vi "Localization FGV.vi"(0 "Action":T1, 1 "Dictionary File Path":path, 5 "VI in":refnum<vi>, 7 "Target Language":string, 9 "UID":string, 11 "error in":errorcluster) -> (6 "Dictionary":T2, 8 "Languages":string[](array[string]), 10 "Translated Word":string, 14 "Current Language":string, 15 "error out":errorcluster)   [LabVIEW 2017, in "JKI Simple Localization.lvlib"]
uses:
  API/JKI Simple Localization.lvlib
  Definitions/Dictionary--Cluster.ctl
  Definitions/Private/Font -- Cluster.ctl
  Definitions/Private/Phrase Dictionary Entry -- Cluster.ctl
  Definitions/Private/Localization FGV Action -- Enum.ctl
  Definitions/Private/VI Info -- Cluster.ctl
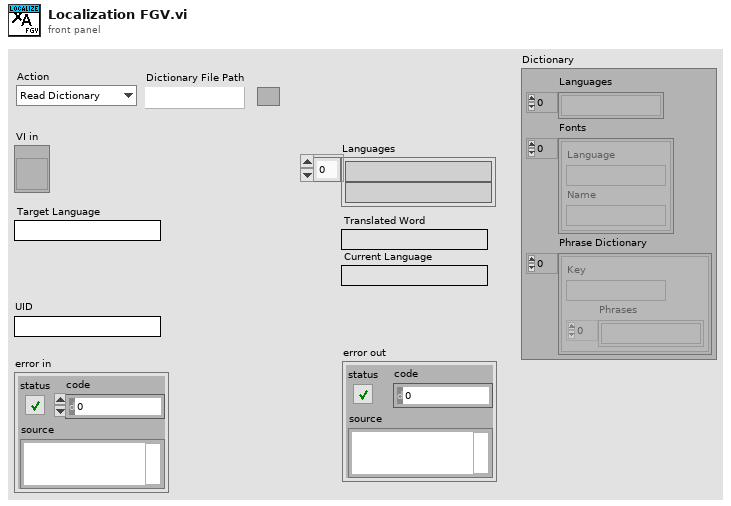
[diagram p1: front panel]
types:
  T1 = typedef "JKI Simple Localization.lvlib/Localization FGV Action -- Enum.ctl" = enum16{"Read Dictionary", "Translate VIs", "Register VI", "Get Languages", "Translate Phrase", "Translate VI", "Unregister"}
  T2 = typedef "JKI Simple Localization.lvlib/Dictionary--Cluster.ctl" = cluster{"Languages":string[], "Fonts":T3[], "Phrase Dictionary":T4[]}
  T3 = typedef "JKI Simple Localization.lvlib/Font -- Cluster.ctl" = cluster{"Language":string, "Name":string}
  T4 = typedef "JKI Simple Localization.lvlib/Phrase Dictionary Entry -- Cluster.ctl" = cluster{"Key":string, "Phrases":string[]}
  T5 = typedef "JKI Simple Localization.lvlib/VI Info -- Cluster.ctl" = cluster{"VI Ref":refnum<vi>, "Language":string}
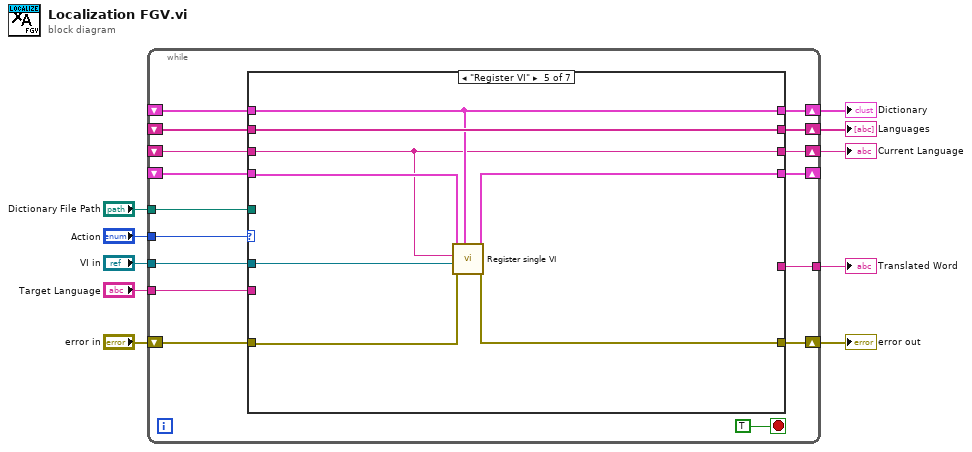
[diagram p0: block diagram]
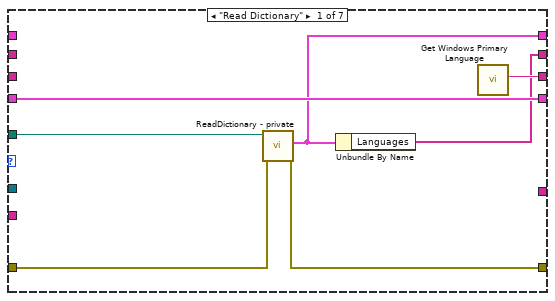
[diagram p2: hidden frame]
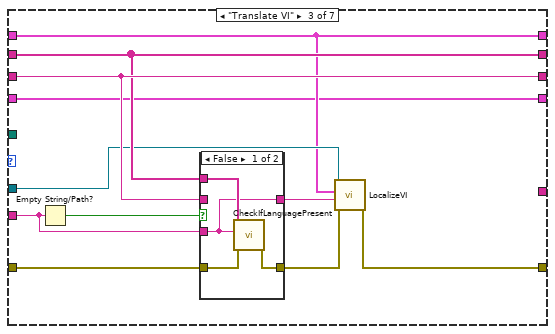
[diagram p4: hidden frame]
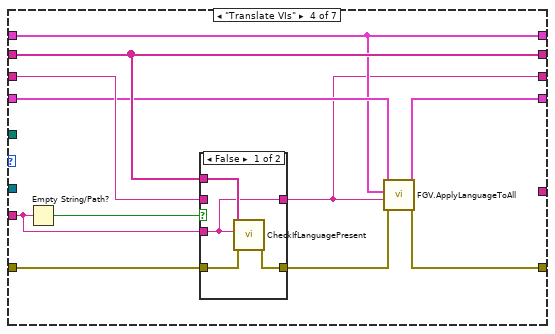
[diagram p6: hidden frame]
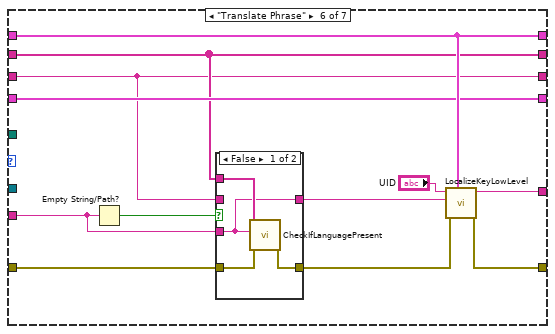
[diagram p8: hidden frame]
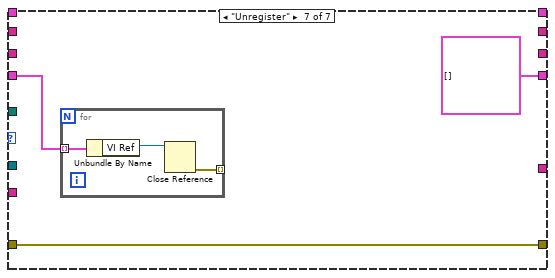
[diagram p10: hidden frame]
diagram:
  n1 = while {
    tunnel: "Action" -> [w25]
    tunnel: "Dictionary File Path" -> [w24]
    shift-right: [w23] -> w1
    shift-left: _ -> [w22]
    shift-right: [w12] -> w9
    shift-left: "error in" -> [w21]
    tunnel: "VI in" -> [w20]
    shift-right: [w19] -> _
    shift-left: _ -> [w18]
    shift-right: [w17] -> w6
    shift-left: _ -> [w16]
    tunnel: "Target Language" -> [w15]
    shift-right: [w14] -> w2
    shift-left: _ -> [w13]
    tunnel: [w11] -> w4
    stop <- TRUE stop-if-true
    n2 = case shown="\"Register VI\"" w25 {
      tunnel: w24 -> [w33 _ _ _ _ _ _]
      tunnel: [w28 w38 w41 w59 w77 w92 _] -> w23
      tunnel: w22 -> [_ w38 w41 w59 w77 w92 _]
      tunnel: w21 -> [w31 w35 w45 w62 w79 w87 w101]
      tunnel: w20 -> [_ _ w42 _ w73 _ _]
      tunnel: [w30 w36 w39 w60 w75 w90 T5[] [] ("VI Status")] -> w19
      tunnel: w18 -> [w30 w36 w39 w61 w76 w90 w100]
      tunnel: [w27 w37 w46 w63 w80 w85 _] -> w17
      tunnel: w16 -> [_ w37 w46 w63 w80 w85 _]
      tunnel: w15 -> [_ _ w47 w64 _ w83 _]
      tunnel: [w29 w34 w48 w56 w74 w82 _] -> w14
      tunnel: w13 -> [_ w34 w48 w65 w74 w82 _]
      tunnel: [w32 w35 w43 w57 w78 w91 w101] -> w12
      tunnel: [_ _ _ _ _ w89 _] -> w11
      frame "Read Dictionary" {
        n3 = call "ReadDictionary - private.vi"("error in (no error)"=w31, "Dictionary File Path"=w33) -> ("error out"=w32:errorcluster, "Dictionary"=w28:T2)  [unwired: 6 in, 2 out]
        n4 = Unbundle By Name(w28) -> ("Languages"=w27:string[])
        n5 = call "Get Windows Primary Language.vi"() -> ("Primary Language"=w29:string)  [unwired: 11 in]
      }
      frame "Get Languages" {
      }
      frame "Translate VI" {
        n6 = Empty String/Path?(string/path=w47) -> (empty?=w49:bool)
        n7 = case shown="False" w49 {
          tunnel: [w51 w54] -> w40
          tunnel: w48 -> [_ w54]
          tunnel: w47 -> [w51 _]
          tunnel: w46 -> [w53 _]
          tunnel: w45 -> [w52 w55]
          tunnel: [w50 w55] -> w44
          frame False {
            n8 = call "CheckIfLanguagePresent.vi"("error in"=w52, "Target Language"=w51, "Languages"=w53) -> ("error out"=w50:errorcluster)  [unwired: 7 in, 1 out]
          }
          frame True {
          }
        }
        n9 = call "LocalizeVI.vi"("error in (no error)"=w44, "Target Language"=w40, "Dictionary"=w41, "VI in"=w42) -> ("error out"=w43:errorcluster)  [unwired: 7 in]
      }
      frame "Translate VIs" {
        n10 = Empty String/Path?(string/path=w64) -> (empty?=w66:bool)
        n11 = case shown="False" w66 {
          tunnel: [w68 w71] -> w56
          tunnel: w65 -> [_ w71]
          tunnel: w64 -> [w68 _]
          tunnel: w63 -> [w70 _]
          tunnel: w62 -> [w69 w72]
          tunnel: [w67 w72] -> w58
          frame False {
            n12 = call "CheckIfLanguagePresent.vi"("error in"=w69, "Target Language"=w68, "Languages"=w70) -> ("error out"=w67:errorcluster)  [unwired: 7 in, 1 out]
          }
          frame True {
          }
        }
        n13 = call "FGV.ApplyLanguageToAll.vi"("error in (no error)"=w58, "Target Language"=w56, "Dictionary"=w59, "VI Status"=w61) -> ("error out"=w57:errorcluster, "VI Status"=w60:T5[])  [unwired: 6 in]
      }
      frame "Register VI" {
        n14 = call "Register single VI.vi"("Dictionary"=w77, "error in (no error)"=w79, "VI in"=w73, "Target Language"=w74, "VI Status"=w76) -> ("Error out"=w78:errorcluster, "VI Status"=w75:T5[])  [unwired: 5 in]
      }
      frame "Translate Phrase" {
        n15 = Empty String/Path?(string/path=w83) -> (empty?=w84:bool)
        n16 = case shown="False" w84 {
          tunnel: [w94 w97] -> w81
          tunnel: w82 -> [_ w97]
          tunnel: w83 -> [w94 _]
          tunnel: w85 -> [w96 _]
          tunnel: w87 -> [w95 w98]
          tunnel: [w93 w98] -> w86
          frame False {
            n17 = call "CheckIfLanguagePresent.vi"("error in"=w95, "Target Language"=w94, "Languages"=w96) -> ("error out"=w93:errorcluster)  [unwired: 7 in, 1 out]
          }
          frame True {
          }
        }
        n18 = call "LocalizeKeyLowLevel.vi"("Dictionary"=w92, "error in (no error)"=w86, "Target Language"=w81, "Key"="UID") -> ("error out"=w91:errorcluster, "Localized Phrase"=w89:string)  [unwired: 6 in]
      }
      frame "Unregister" {
        n19 = for {
          tunnel: w100 -> [w104] mode=indexing
          tunnel: [w102] -> _ mode=indexing
          n20 = Unbundle By Name(w104) -> ("VI Ref"=w103:refnum<vi>)
          n21 = Close Reference(reference=w103) -> (error out=w102:errorcluster)  [unwired: 1 in]
        }
      }
    }
  }
  "error out" <- w9
  "Dictionary" <- w1
  "Languages" <- w6
  "Translated Word" <- w4
  "Current Language" <- w2
